vi "Red_Green.vi"(8 "error in (no error)":errorcluster, 11 "Refnum in":T1) -> (0 "error out":errorcluster, 3 "Refnum out":T1)   [LabVIEW 2018]
uses:
  <vilib>/vision/Image Controls.llb/IMAQ Image.ctl
  <vilib>/vision/NI_Vision_Development_Module.lvlib
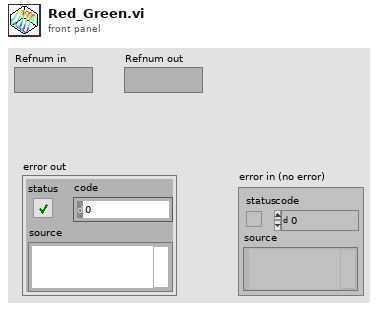
[diagram p1: front panel]
types:
  T1 = typedef "IMAQ Image.ctl" = refnum<image>
  T2 = typedef "Image Type" = u32
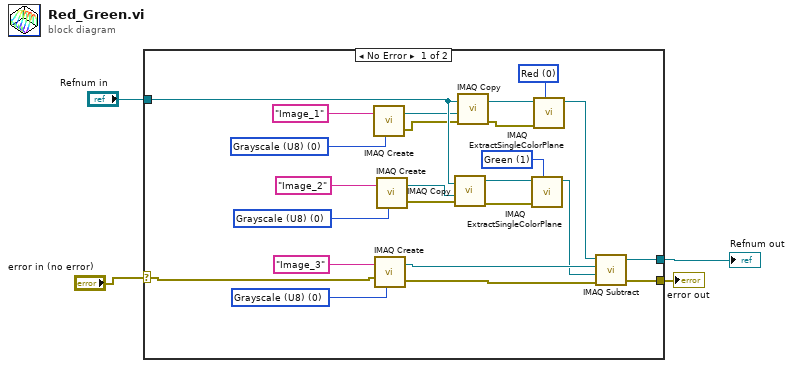
[diagram p0: block diagram]
diagram:
  n1 = case shown="No Error" "error in (no error)" {
    selector: "error in (no error)" -> [w6 w30]
    tunnel: "Refnum in" -> [w28 w29]
    tunnel: [w7 w29] -> w3
    tunnel: [w5 w30] -> w1
    frame No Error {
      w22 = T2 0 items=["Grayscale (U8)", "Grayscale (I16)", "Grayscale (SGL)", "Complex (CSG)", "RGB (U32)", "HSL (U32)", "RGB (U64)", "Grayscale (U16)"] ("Image Type")
      w16 = 1 items=["Red", "Green", "Blue", "Hue", "Saturation", "Luminance", "Value", "Intensity"] ("Color Plane")
      w14 = 0 items=["Red", "Green", "Blue", "Hue", "Saturation", "Luminance", "Value", "Intensity"] ("Color Plane")
      w11 = T2 0 items=["Grayscale (U8)", "Grayscale (I16)", "Grayscale (SGL)", "Complex (CSG)", "RGB (U32)", "HSL (U32)", "RGB (U64)", "Grayscale (U16)"] ("Image Type")
      w9 = T2 0 items=["Grayscale (U8)", "Grayscale (I16)", "Grayscale (SGL)", "Complex (CSG)", "RGB (U32)", "HSL (U32)", "RGB (U64)", "Grayscale (U16)"] ("Image Type")
      n2 = call "IMAQ Create"("Image Name"="Image_1", "Image Type"=w9) -> ("New Image"=w10:T1, "error out"=w26:errorcluster)  [unwired: 3 in]
      n3 = call "IMAQ Create"("Image Name"="Image_3", "Image Type"=w22, "error in (no error)"=w6) -> ("New Image"=w23:T1, "error out"=w24:errorcluster)  [unwired: 2 in]
      n4 = call "IMAQ Create"("Image Name"="Image_2", "Image Type"=w11) -> ("New Image"=w13:T1, "error out"=w25:errorcluster)  [unwired: 3 in]
      n5 = call "IMAQ Copy"("error in (no error)"=w25, "Image Dst"=w13, "Image Src"=w28) -> ("error out"=w18:errorcluster, "Image Dst Out"=w15:T1)  [unwired: 3 in]
      n6 = call "IMAQ Copy"("error in (no error)"=w26, "Image Dst"=w10, "Image Src"=w28) -> ("error out"=w17:errorcluster, "Image Dst Out"=w27:T1)  [unwired: 3 in]
      n7 = call "IMAQ ExtractSingleColorPlane"("Color Plane"=w16, "error in (no error)"=w18, "Image Src"=w15) -> ("Image Dst Out"=w20:T1)  [unwired: 7 in, 1 out]
      n8 = call "IMAQ ExtractSingleColorPlane"("Color Plane"=w14, "error in (no error)"=w17, "Image Src"=w27) -> ("Image Dst Out"=w19:T1)  [unwired: 7 in, 1 out]
      n9 = call "IMAQ Subtract"("Image Src A"=w19, "Image Dst"=w23, "Image Src B"=w20, "error in (no error)"=w24) -> ("Image Dst Out"=w7:T1, "error out"=w5:errorcluster)  [unwired: 3 in]
    }
    frame Error {
    }
  }
  "Refnum out" <- w3
  "error out" <- w1
